vi "Log Table.vi"(8 "Error in":errorcluster, 9 "Catalog ID":T1, 10 "Time":T2, 11 "Date":T3) -> (0 "Error out":errorcluster, 3 "Log Table":string[][](array[string]))   [LabVIEW 2020, in "Database Lib.lvlib"]
uses:
  Database Lib.lvlib
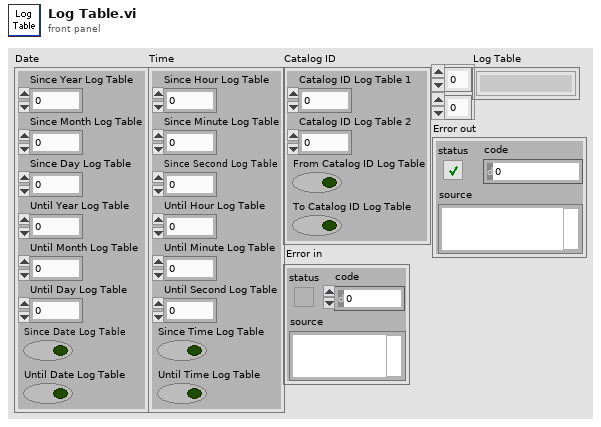
[diagram p1: front panel]
types:
  T1 = cluster{"Catalog ID Log Table 1":u16, "Catalog ID Log Table 2":u16, "From Catalog ID Log Table":bool, "To Catalog ID Log Table":bool}
  T2 = cluster{"Since Hour Log Table":u8, "Since Minute Log Table":u8, "Since Second Log Table":u8, "Until Hour Log Table":u8, "Until Minute Log Table":u8, "Until Second Log Table":u8, "Since Time Log Table":bool, "Until Time Log Table":bool}
  T3 = cluster{"Since Year Log Table":u16, "Since Month Log Table":u8, "Since Day Log Table":u8, "Until Year Log Table":u16, "Until Month Log Table":u8, "Until Day Log Table":u8, "Since Date Log Table":bool, "Until Date Log Table":bool}
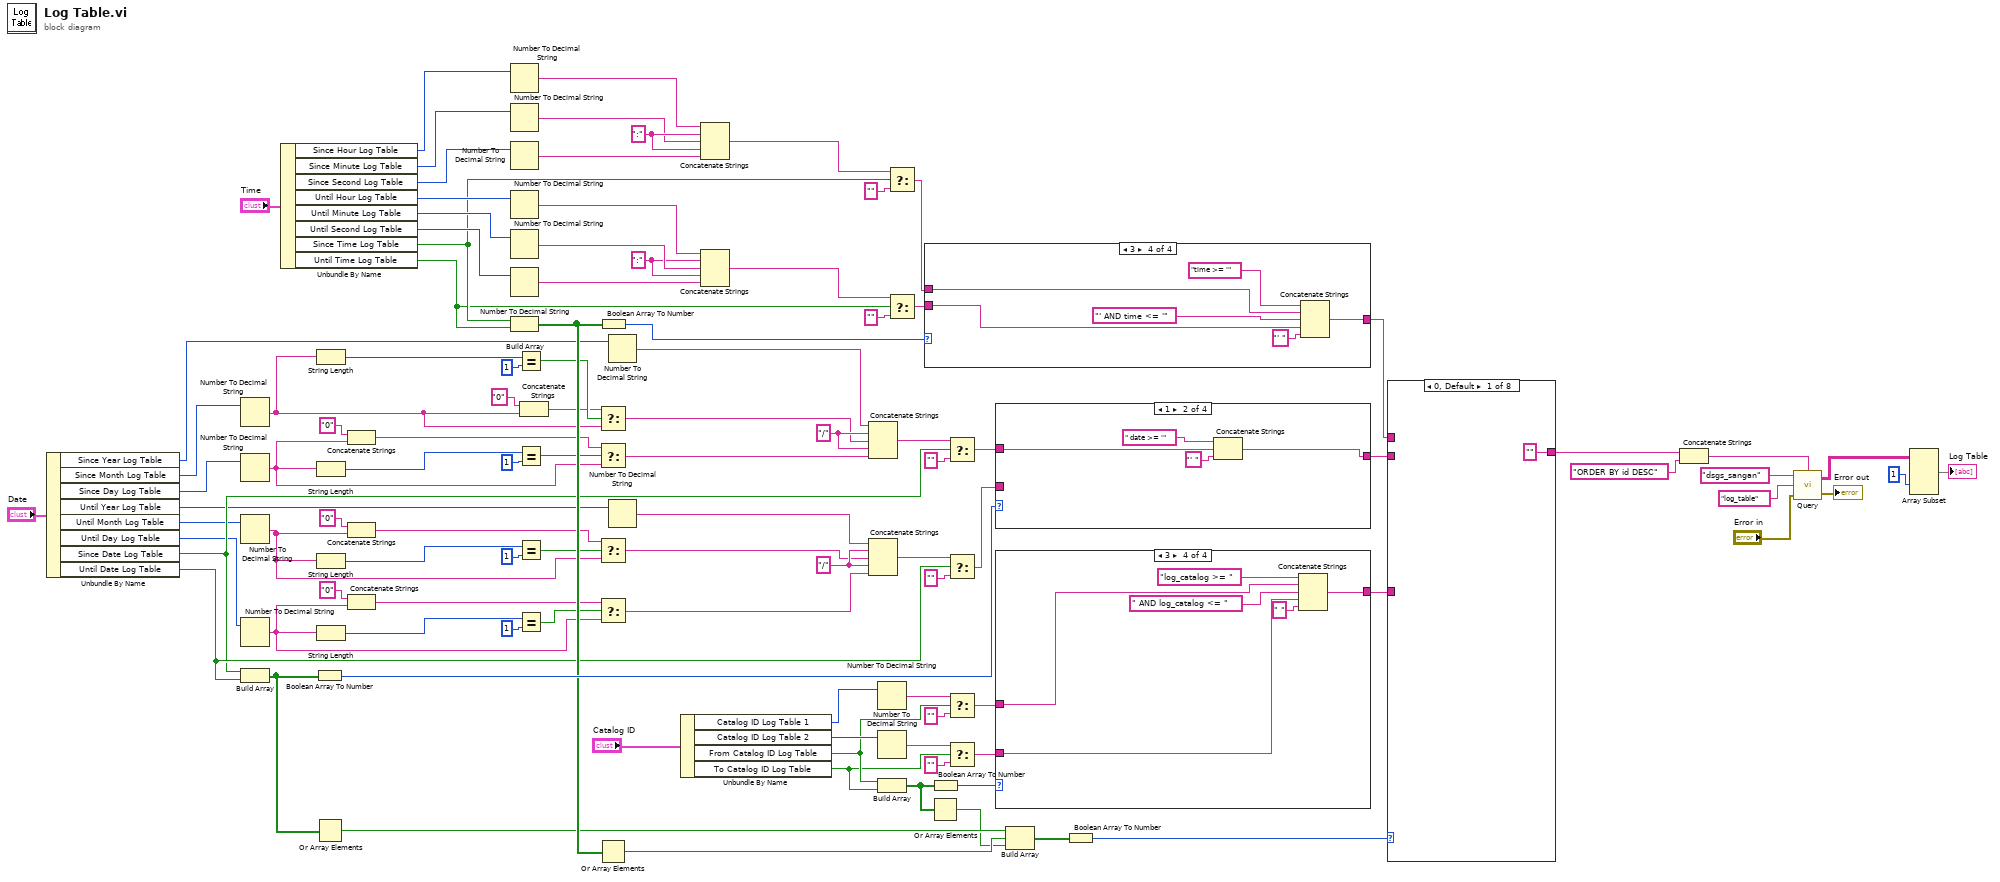
[diagram p0: block diagram]
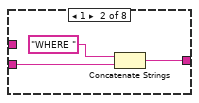
[diagram p2: hidden frame]
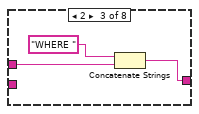
[diagram p3: hidden frame]
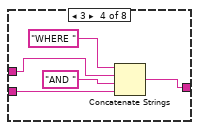
[diagram p4: hidden frame]
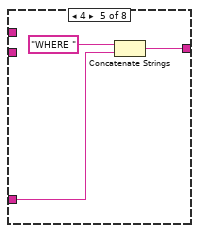
[diagram p5: hidden frame]
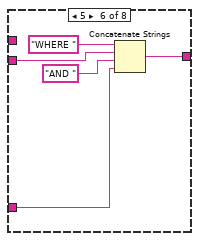
[diagram p6: hidden frame]
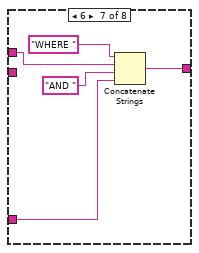
[diagram p7: hidden frame]
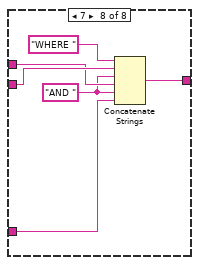
[diagram p8: hidden frame]
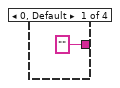
[diagram p9: hidden frame]
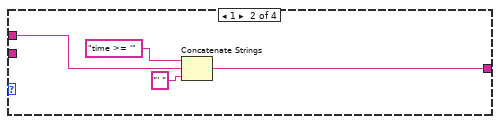
[diagram p10: hidden frame]
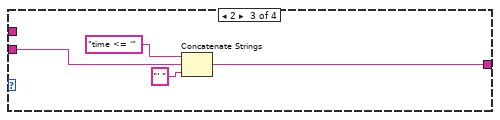
[diagram p11: hidden frame]
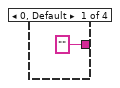
[diagram p12: hidden frame]
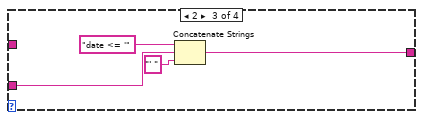
[diagram p13: hidden frame]
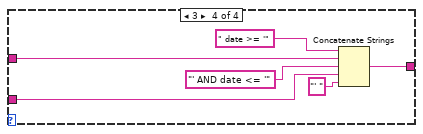
[diagram p14: hidden frame]
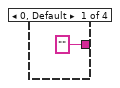
[diagram p15: hidden frame]
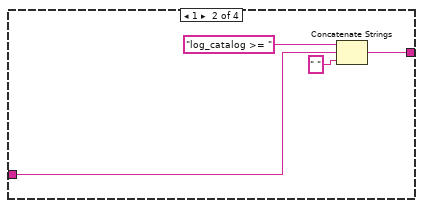
[diagram p16: hidden frame]
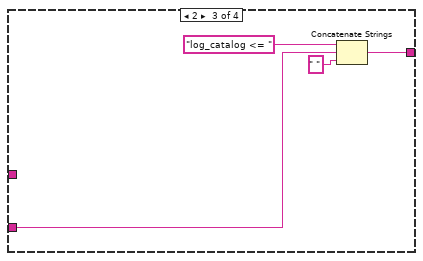
[diagram p17: hidden frame]
diagram:
  w86 = "/" ("string")
  w90 = ":" ("string")
  w104 = ":" ("string")
  w105 = "/" ("string")
  n1 = Unbundle By Name("Date") -> ("Since Year Log Table"=w16:u16, "Since Month Log Table"=w13:u8, "Since Day Log Table"=w12:u8, "Until Year Log Table"=w11:u16, "Until Month Log Table"=w10:u8, "Until Day Log Table"=w9:u8, "Since Date Log Table"=w14:bool, "Until Date Log Table"=w15:bool)
  n2 = Number To Decimal String(number=w13) -> (decimal integer string=w46:string)  [unwired: 1 in]
  n3 = Number To Decimal String(number=w12) -> (decimal integer string=w43:string)  [unwired: 1 in]
  n4 = Number To Decimal String(number=w10) -> (decimal integer string=w30:string)  [unwired: 1 in]
  n5 = Number To Decimal String(number=w9) -> (decimal integer string=w29:string)  [unwired: 1 in]
  n6 = Build Array(w14, w15) -> (w69:bool[])
  n7 = Unbundle By Name("Time") -> ("Since Hour Log Table"=w25:u8, "Since Minute Log Table"=w24:u8, "Since Second Log Table"=w23:u8, "Until Hour Log Table"=w20:u8, "Until Minute Log Table"=w21:u8, "Until Second Log Table"=w22:u8, "Since Time Log Table"=w19:bool, "Until Time Log Table"=w18:bool)
  n8 = Boolean Array To Number(Boolean array=w69) -> (number=w76:u32)
  n9 = Or Array Elements(Boolean array=w69) -> (logical OR=w67:bool)
  n10 = String Length(string=w46) -> (length=w54:i32)
  n11 = String Length(string=w43) -> (length=w51:i32)
  n12 = String Length(string=w30) -> (length=w31:i32)
  n13 = String Length(string=w29) -> (length=w34:i32)
  n14 = Concatenate Strings("0" ("string"), w43) -> (w44:string)
  n15 = Concatenate Strings("0" ("string"), w30) -> (w38:string)
  n16 = Concatenate Strings("0" ("string"), w29) -> (w40:string)
  n17 = Number To Decimal String(number=w25) -> (decimal integer string=w103:string)  [unwired: 1 in]
  n18 = Number To Decimal String(number=w24) -> (decimal integer string=w102:string)  [unwired: 1 in]
  n19 = Number To Decimal String(number=w23) -> (decimal integer string=w101:string)  [unwired: 1 in]
  n20 = Number To Decimal String(number=w20) -> (decimal integer string=w91:string)  [unwired: 1 in]
  n21 = Number To Decimal String(number=w21) -> (decimal integer string=w92:string)  [unwired: 1 in]
  n22 = Number To Decimal String(number=w22) -> (decimal integer string=w89:string)  [unwired: 1 in]
  n23 = Build Array(w19, w18) -> (w68:bool[])
  n24 = Equal?(x=w54, y=1) -> (x = y?=w50:bool)
  n25 = Equal?(x=w51, y=1) -> (x = y?=w49:bool)
  n26 = Equal?(x=w31, y=1) -> (x = y?=w35:bool)
  n27 = Equal?(x=w34, y=1) -> (x = y?=w36:bool)
  n28 = Concatenate Strings("0" ("string"), w46) -> (w47:string)
  n29 = Select(t=w47, s=w50, f=w46) -> (s? t:f=w42:string)
  n30 = Select(t=w44, s=w49, f=w43) -> (s? t:f=w41:string)
  n31 = Select(t=w38, s=w35, f=w30) -> (s? t:f=w27:string)
  n32 = Select(t=w40, s=w36, f=w29) -> (s? t:f=w28:string)
  n33 = Or Array Elements(Boolean array=w68) -> (logical OR=w66:bool)
  n34 = Boolean Array To Number(Boolean array=w68) -> (number=w73:u32)
  n35 = Number To Decimal String(number=w16) -> (decimal integer string=w100:string)  [unwired: 1 in]
  n36 = Number To Decimal String(number=w11) -> (decimal integer string=w87:string)  [unwired: 1 in]
  n37 = Unbundle By Name("Catalog ID") -> ("Catalog ID Log Table 1"=w7:u16, "Catalog ID Log Table 2"=w6:u16, "From Catalog ID Log Table"=w5:bool, "To Catalog ID Log Table"=w4:bool)
  n38 = Concatenate Strings(w103, w104, w102, w104, w101) -> (w97:string)
  n39 = Concatenate Strings(w91, w90, w92, w90, w89) -> (w94:string)
  n40 = Concatenate Strings(w100, w105, w42, w105, w41) -> (w56:string)
  n41 = Concatenate Strings(w87, w86, w27, w86, w28) -> (w55:string)
  n42 = Number To Decimal String(number=w7) -> (decimal integer string=w96:string)  [unwired: 1 in]
  n43 = Number To Decimal String(number=w6) -> (decimal integer string=w84:string)  [unwired: 1 in]
  n44 = Build Array(w5, w4) -> (w70:bool[])
  n45 = Select(t=w97, s=w19, f="") -> (s? t:f=w72:string)
  n46 = Select(t=w94, s=w18, f="") -> (s? t:f=w71:string)
  n47 = case shown="3" w73 {
    tunnel: ["" ("f") w108 w113 w116] -> w61
    tunnel: w72 -> [_ w109 _ w119]
    tunnel: w71 -> [_ _ w112 w117]
    frame 0, Default {
    }
    frame 1 {
      n48 = Concatenate Strings("time >= '" ("f"), w109, "' " ("string")) -> (w108:string)
    }
    frame 2 {
      n49 = Concatenate Strings("time <= '" ("f"), w112, "' " ("string")) -> (w113:string)
    }
    frame 3 {
      n50 = Concatenate Strings("time >= '" ("f"), w119, "' AND time <= '" ("string"), w117, "' " ("string")) -> (w116:string)
    }
  }
  n51 = Or Array Elements(Boolean array=w70) -> (logical OR=w65:bool)
  n52 = Boolean Array To Number(Boolean array=w70) -> (number=w83:u32)
  n53 = Select(t=w56, s=w14, f="") -> (s? t:f=w75:string)
  n54 = Select(t=w55, s=w15, f="") -> (s? t:f=w74:string)
  n55 = Select(t=w96, s=w5, f="") -> (s? t:f=w82:string)
  n56 = Select(t=w84, s=w4, f="") -> (s? t:f=w81:string)
  n57 = case shown="1" w76 {
    tunnel: ["" ("f") w123 w128 w131] -> w62
    tunnel: w75 -> [_ w124 _ w134]
    tunnel: w74 -> [_ _ w127 w132]
    frame 0, Default {
    }
    frame 1 {
      n58 = Concatenate Strings(" date >= '" ("f"), w124, "' " ("string")) -> (w123:string)
    }
    frame 2 {
      n59 = Concatenate Strings("date <= '" ("f"), w127, "' " ("string")) -> (w128:string)
    }
    frame 3 {
      n60 = Concatenate Strings(" date >= '" ("f"), w134, "' AND date <= '" ("string"), w132, "' " ("string")) -> (w131:string)
    }
  }
  n61 = case shown="3" w83 {
    tunnel: ["" ("f") w138 w143 w146] -> w60
    tunnel: w82 -> [_ w139 _ w149]
    tunnel: w81 -> [_ _ w142 w147]
    frame 0, Default {
    }
    frame 1 {
      n62 = Concatenate Strings("log_catalog >= " ("f"), w139, " " ("string")) -> (w138:string)
    }
    frame 2 {
      n63 = Concatenate Strings("log_catalog <= " ("f"), w142, " " ("string")) -> (w143:string)
    }
    frame 3 {
      n64 = Concatenate Strings("log_catalog >= " ("f"), w149, " AND log_catalog <= " ("string"), w147, " " ("string")) -> (w146:string)
    }
  }
  n65 = Build Array(w67, w66, w65) -> (w64:bool[])
  n66 = Boolean Array To Number(Boolean array=w64) -> (number=w63:u32)
  n67 = case shown="0, Default" w63 {
    tunnel: ["" ("f") w154 w156 w158 w163 w166 w171 w176] -> w59
    tunnel: w62 -> [_ w152 _ w159 _ w169 _ w180]
    tunnel: w61 -> [_ _ w155 w161 _ _ w173 w179]
    tunnel: w60 -> [_ _ _ _ w164 w167 w172 w177]
    frame 0, Default {
    }
    frame 1 {
      n68 = Concatenate Strings("WHERE " ("f"), w152) -> (w154:string)
    }
    frame 2 {
      n69 = Concatenate Strings("WHERE " ("f"), w155) -> (w156:string)
    }
    frame 3 {
      n70 = Concatenate Strings("WHERE " ("f"), w161, "AND " ("string"), w159) -> (w158:string)
    }
    frame 4 {
      n71 = Concatenate Strings("WHERE " ("f"), w164) -> (w163:string)
    }
    frame 5 {
      n72 = Concatenate Strings("WHERE " ("f"), w169, "AND " ("string"), w167) -> (w166:string)
    }
    frame 6 {
      n73 = Concatenate Strings("WHERE " ("f"), w173, "AND " ("string"), w172) -> (w171:string)
    }
    frame 7 {
      w178 = "AND " ("string")
      n74 = Concatenate Strings("WHERE " ("f"), w180, w178, w179, w178, w177) -> (w176:string)
    }
  }
  n75 = Concatenate Strings(w59, "ORDER BY id DESC" ("string")) -> (w79:string)
  n76 = call "Query.vi"("Condition"=w79, "Error in"="Error in", "Table Name"="log_table", "Connection Name"="dsgs_sangan") -> ("Error out"=→"Error out":errorcluster, "data"=w58:string[][])
  n77 = Array Subset(array=w58, index (col)=1 ("index")) -> (→"Log Table":string[][])  [unwired: 3 in]
